vi "上升下降沿.vi"(5 "初始化":bool, 9 "输入数据":bool) -> (3 "上升下降沿":bool)   [LabVIEW 2012, in "边沿检测.lvlib"]
uses:
  <vilib>/ptbypt/NI_PtbyPt.lvlib
panel:
  out "下降沿":bool
  out "上升沿":bool
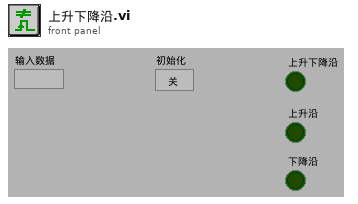
[diagram p1: front panel]
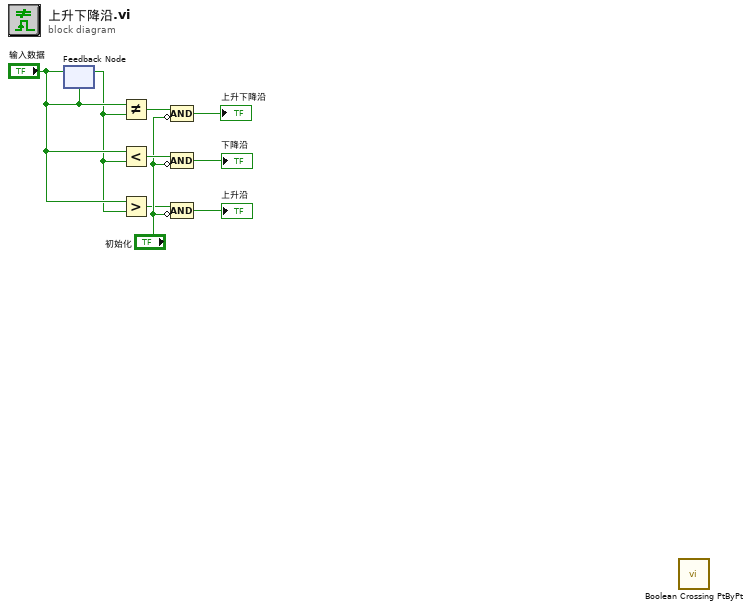
[diagram p0: block diagram]
diagram:
  n1 = feedback-in #1("输入数据") -> ()
  n2 = feedback #1("输入数据") -> (w7:bool)
  n3 = Not Equal?(x="输入数据", y=w7) -> (x != y?=w6:bool)
  n4 = Less?(x="输入数据", y=w7) -> (x < y?=w9:bool)
  n5 = Greater?(x="输入数据", y=w7) -> (0:w3:bool)
  n6 = Compound Arithmetic op=AND(w6, invert "初始化") -> (→"上升下降沿":bool)
  n7 = Compound Arithmetic op=AND(w9, invert "初始化") -> (→"下降沿":bool)
  n8 = Compound Arithmetic op=AND(w3, invert "初始化") -> (→"上升沿":bool)
  n9 = call <vilib>:"Boolean Crossing PtByPt.vi"() -> ()  [unwired: 3 in, 1 out]
